vi "ReadVoltCurr.vi"(6 "time out":u32, 10 "类型":u32(ring)=4 items=["PCI5121"=1, "PCI9810"=2, "USBCAN1"=3, "USBCAN2"=4, "PCI9820"=5, "CAN232"=6, "PCI5110"=7, "CANLite(mini)"=8, "ISA9620"=9, "ISA5420"=10, "PC104CAN"=11, "CANET"=17, "DNP9810"=13, "USBCAN-E-U"=20, "USBCAN-2E-U"=21], 12 "设备索引":u32(ring) items=["0", "1", "2", "3", "4", "5", "6", "7", "8", "9", "10", "11", "12", "13", "14", "15", ""], 16 "CAN路数":u32(ring) items=["0", "1"]) -> (20 "recv ok?":bool, 21 "InSumv":dbl, 22 "OutSumv":dbl, 23 "InstantCurr":dbl, 24 "AvgCurr":dbl)   [LabVIEW 2013]
uses:
  AutoBurn/Settings/ControlCAN.dll
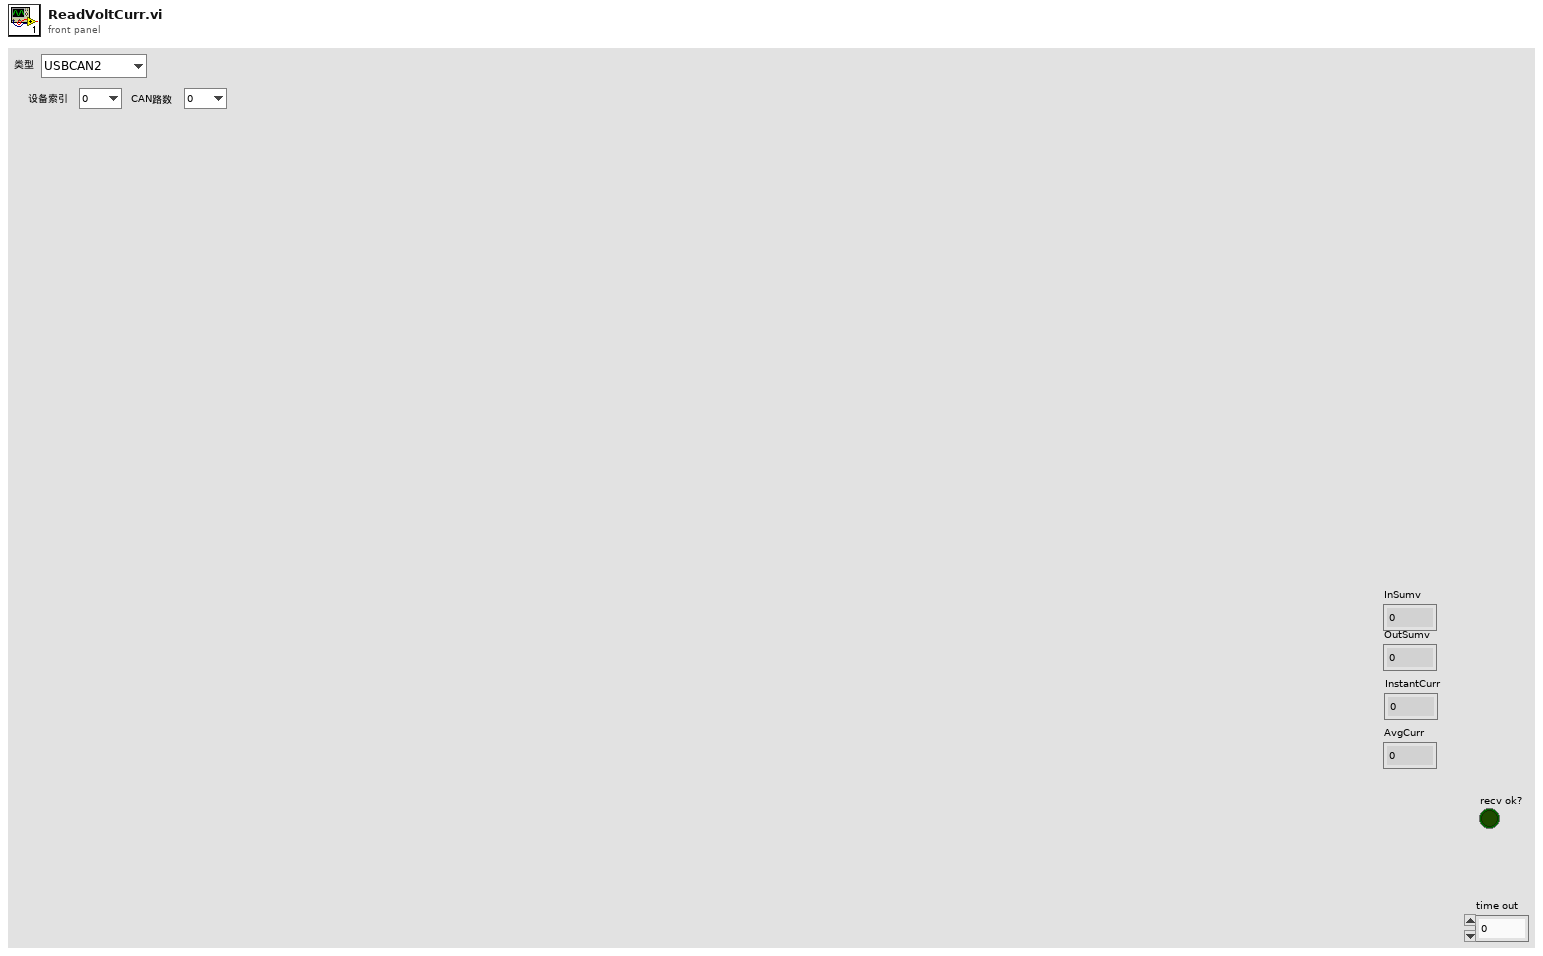
[diagram p1: front panel]
types:
  T1 = cluster{"ID":u32, "TimeStamp":u32, "TimeFlag":u8, "SendType":u8, "RemoteFlag":u8, "ExternFlag":u8, "DataLen":u8, u8, u8, u8, u8, u8, u8, u8, u8, u8, u8, u8}
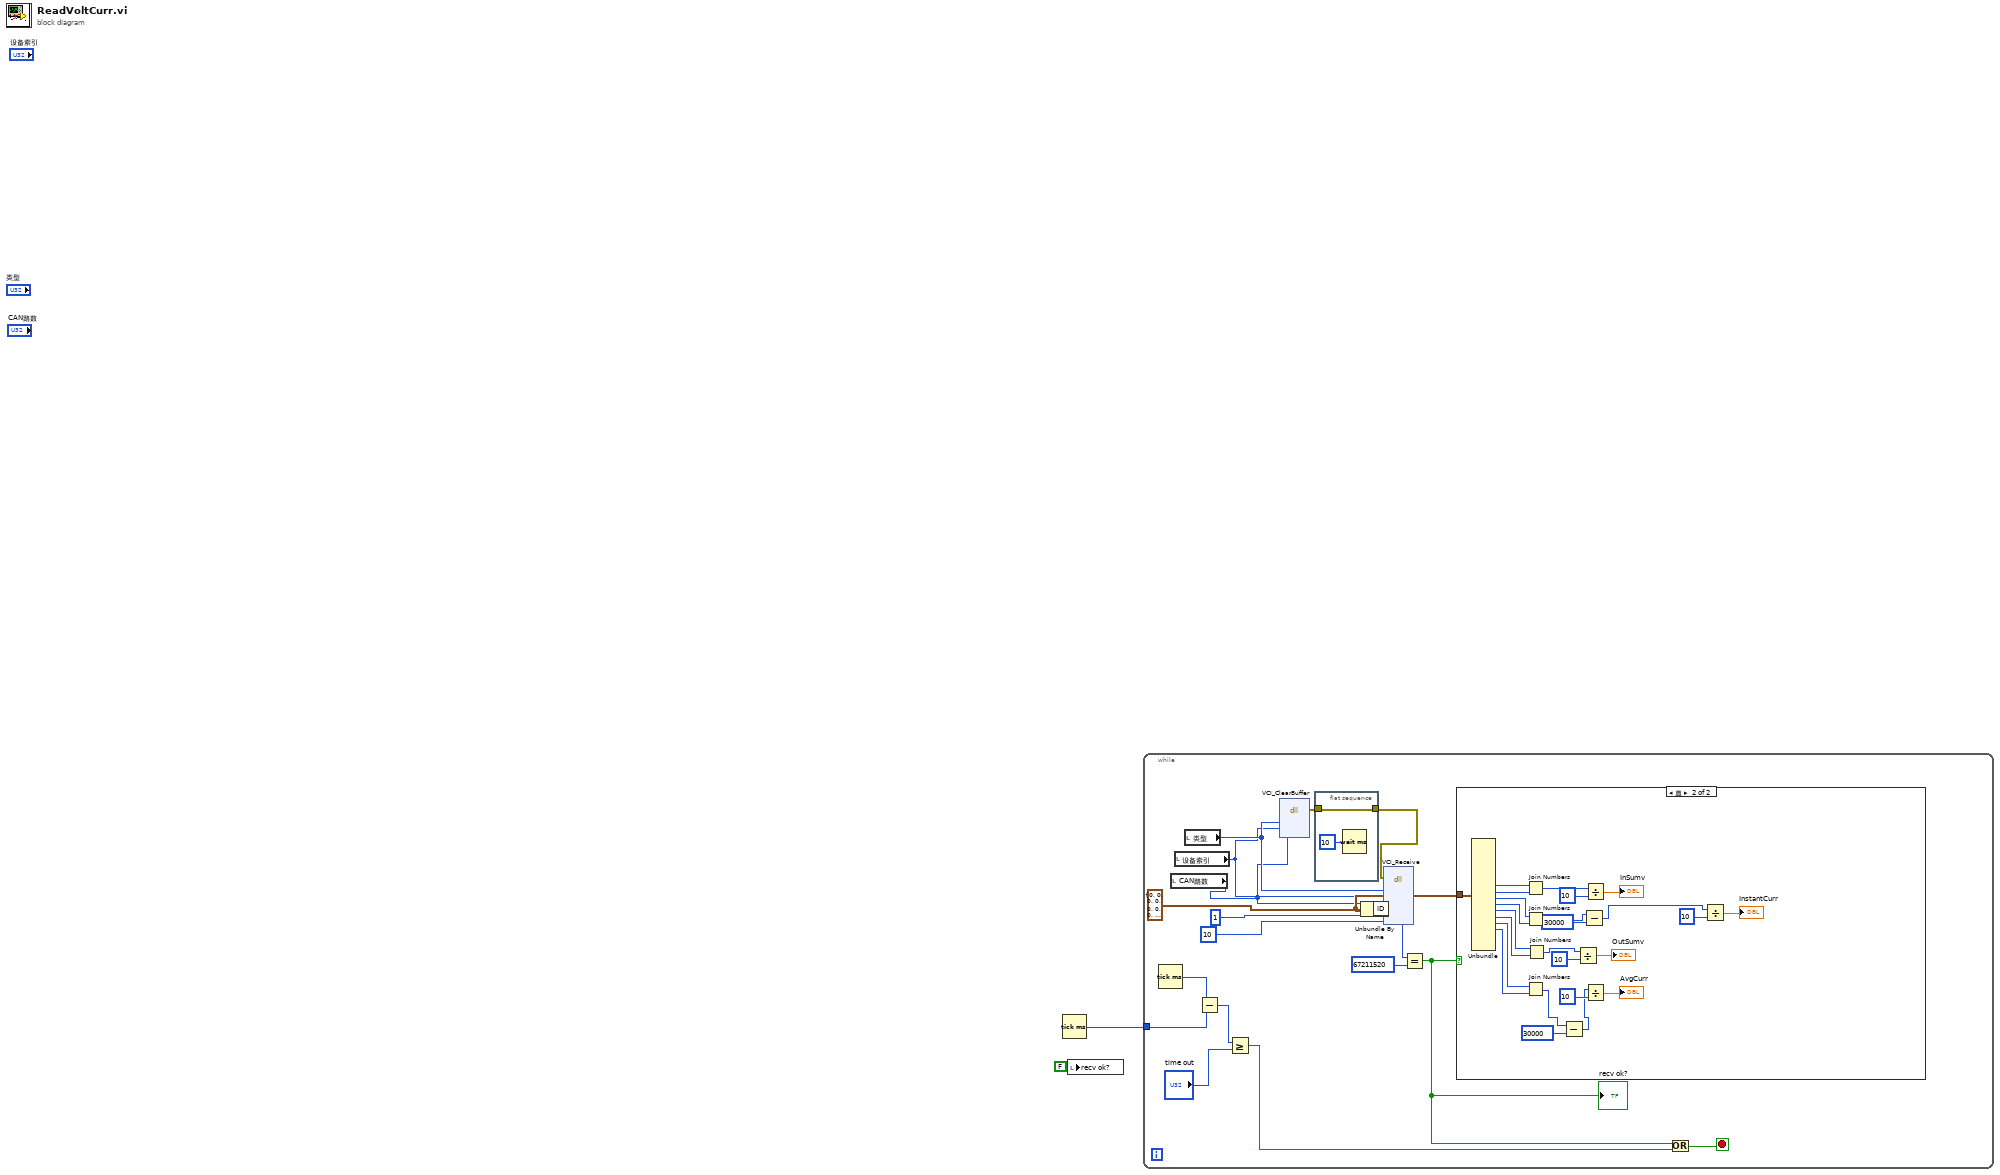
[diagram p0: block diagram]
diagram:
  n1 = Tick Count (ms)() -> (millisecond timer value=w2:u32)
  n2 = local write "recv ok?"(FALSE ("x = y?")) -> ()
  n3 = while {
    tunnel: w2 -> [w16]
    stop <- w10 stop-if-true
    n4 = Tick Count (ms)() -> (millisecond timer value=w17:u32)
    n5 = local read "CAN路数"() -> (w5:u32)
    n6 = local read "设备索引"() -> (w6:u32)
    n7 = local read "类型"() -> (w7:u32)
    n8 = Subtract(x=w17, y=w16) -> (x-y=w15:u32)
    n9 = Greater Or Equal?(x=w15, y="time out") -> (x >= y?=w11:bool)
    n10 = dll-call lib="F:/Bluewave New Energy/SVN_Work/AutoTest_TestStand/trunk/AutoTest_TestStand/Driver/ZlgCan/BHN01/AutoBurn/Settings/ControlCAN.dll" fn="VCI_ClearBuffer" label="VCI_Clearbuffer"("DeviceType"=w7, "DeviceInd"=w6, "CANInd"=w5) -> (error out=w3:errorcluster)  [unwired: 4 in, 4 out]
    n11 = flat-sequence {
      tunnel: [w22] -> w4
      tunnel: w3 -> [w22]
      frame #0 {
        n12 = Wait (ms)(milliseconds to wait=u32 10 ("等待时间（毫秒）")) -> ()  [unwired: 1 out]
      }
    }
    n13 = dll-call lib="F:/Bluewave New Energy/SVN_Work/AutoTest_TestStand/trunk/AutoTest_TestStand/Driver/ZlgCan/BHN01/AutoBurn/Settings/ControlCAN.dll" fn="VCI_Receive"(error in=w4, "DeviceType"=w7, "DeviceInd"=w6, "CANInd"=w5, "pReceive"=T1 {"ID"=0, "TimeStamp"=0, "TimeFlag"=0, "SendType"=0, "RemoteFlag"=0, "ExternFlag"=0, "DataLen"=0, 0, 0, 0, 0, 0, 0, 0, 0, 0, 0, 0}, "Len"=u32 1, "WaitTime"=10) -> ("pReceive"=w9:T1)  [unwired: 7 in, 3 out]
    n14 = Unbundle By Name(w9) -> ("ID"=w13:u32)
    n15 = Equal?(x=w13, y=u32 67211520) -> (x = y?=w12:bool)
    "recv ok?" <- w12
    n16 = case shown="真" w12 {
      tunnel: w9 -> [_ w47]
      frame False {
      }
      frame True {
        n17 = Unbundle(w47) -> (w46:u8, w45:u8, w35:u8, w34:u8, w33:u8, w32:u8, w31:u8, w30:u8)  [unwired: 10 out]
        n18 = Join Numbers(hi=w46, lo=w45) -> ((hi.lo)=w44:u16)
        n19 = Join Numbers(hi=w35, lo=w34) -> ((hi.lo)=w28:u16)
        n20 = Join Numbers(hi=w31, lo=w30) -> ((hi.lo)=w24:u16)
        n21 = Join Numbers(hi=w33, lo=w32) -> ((hi.lo)=w29:u16)
        n22 = Subtract(x=w24, y=u16 30000) -> (x-y=w23:u16)
        n23 = Divide(x=w29, y=u16 10) -> (x/y=→"OutSumv":dbl)
        n24 = Subtract(x=w28, y=u16 30000) -> (x-y=w26:u16)
        n25 = Divide(x=w44, y=u16 10) -> (x/y=→"InSumv":dbl)
        n26 = Divide(x=w23, y=u16 10) -> (x/y=→"AvgCurr":dbl)
        n27 = Divide(x=w26, y=u16 10) -> (x/y=→"InstantCurr":dbl)
      }
    }
    n28 = Or(x=w12, y=w11) -> (x .or. y?=w10:bool)
  }
